vi "SYST_COMM_GPIB_RDEV_READ.vi"(0 "VISA IN":refnum<visa-resource-name>, 5 "error in":errorcluster, 7 "ID":i32, 9 "Delay Time (s)":dbl=1.0) -> (14 "VISA Out":refnum<visa-resource-name>, 16 "Data":string, 19 "error out":errorcluster)   [LabVIEW 2018, in "PNA-X.lvlib"]
doc: "SYSTem:COMMunicate:GPIB:RDEVice:READ? <ID> \n1870\n\n(Read-only) Returns data from the GPIB pass-through device. \nParameters \n<ID> Session identification number that was returned with the OPEN? command. \nExamples See an example program \nReturn Type String \nDefault Not Applicable"
uses:
  PNA-X.lvlib
  Instance           1 32Saved   SYST_COMM_GPIB_RDEV_READ .vi
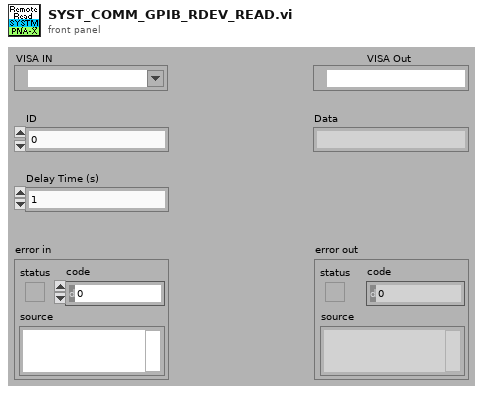
[diagram p1: front panel]
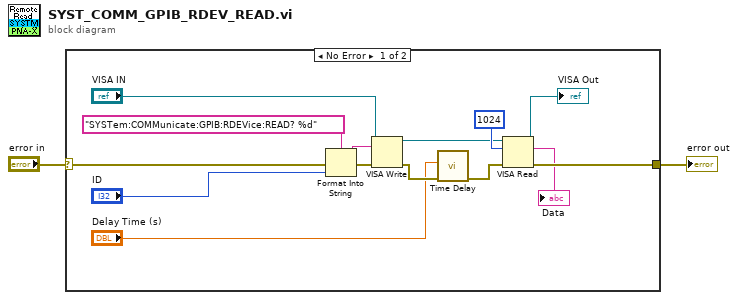
[diagram p0: block diagram]
diagram:
  n1 = case shown="No Error" "error in" {
    selector: "error in" -> [w16 w17]
    tunnel: [w9 w17] -> w1
    frame No Error {
      n2 = Format Into String(format string="SYSTem:COMMunicate:GPIB:RDEVice:READ? %d" ("Cmdline"), error in=w16, "ID") -> (resulting string=w14:string, error out=w15:errorcluster)  [unwired: 1 in]
      n3 = VISA Write(VISA resource name="VISA IN", write buffer=w14, error in (no error)=w15) -> (VISA resource name out=w10:refnum<visa-resource-name>, error out=w5:errorcluster)  [unwired: 1 out]
      n4 = call "Time Delay"("error in (no error)"=w5, "Delay Time (s)"="Delay Time (s)") -> ("error out"=w4:errorcluster)  [unwired: 9 in]
      n5 = VISA Read(VISA resource name=w10, byte count=1024, error in (no error)=w4) -> (VISA resource name out=→"VISA Out":refnum<visa-resource-name>, read buffer=→"Data":string, error out=w9:errorcluster)  [unwired: 1 out]
    }
    frame Error {
    }
  }
  "error out" <- w1
